vi "Read Status String.vi"(8 "error in (no error)":errorcluster, 11 "Update Status Display in":refnum<class "Update Status Display.lvclass">) -> (0 "error out":errorcluster, 2 "Status String":string, 3 "Update Status Display out":refnum<class "Update Status Display.lvclass">)   [LabVIEW 2015, in "Generic UI Actor.lvlib" / "Update Status Display.lvclass"]
uses:
  Update Status Display.lvclass
  Update Status Display.lvclass/Update Status Display.ctl
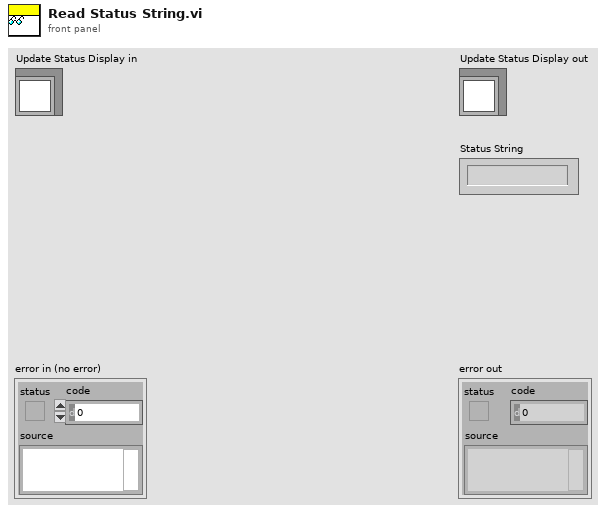
[diagram p1: front panel]
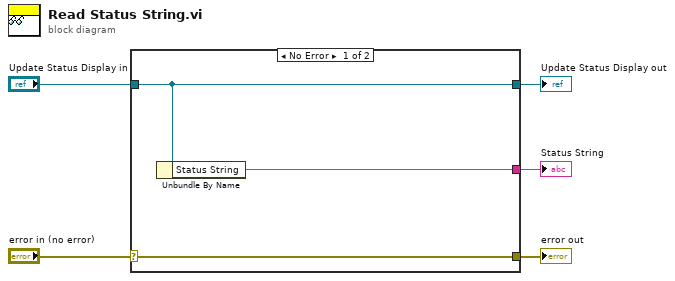
[diagram p0: block diagram]
diagram:
  n1 = case shown="No Error" "error in (no error)" {
    selector: "error in (no error)" -> [w8 w9]
    tunnel: [w8 w9] -> w4
    tunnel: [w7 w10] -> w2
    tunnel: "Update Status Display in" -> [w7 w10]
    tunnel: [w6 _] -> w1
    frame No Error {
      n2 = Unbundle By Name(w7) -> ("Status String"=w6:string)
    }
    frame Error {
    }
  }
  "error out" <- w4
  "Update Status Display out" <- w2
  "Status String" <- w1
